vi "Remove by Name.vi"(8 "error in (no error)":errorcluster, 11 "buffer_name":string="/example") -> (0 "error out":errorcluster)   [LabVIEW 2021, in "CIF_NI_CIPC.lvlib"]
doc: "Removes a CIPC buffer from the system."
uses:
  CIF_NI_CIPC.lvlib
  <vilib>/Utility/error.llb/Trim Whitespace.vi
  <vilib>/Utility/error.llb/Error Cluster From Error Code.vi
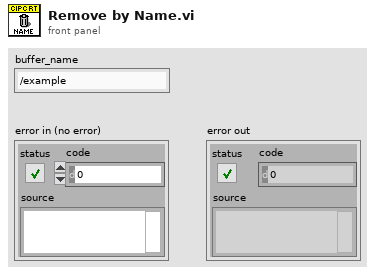
[diagram p1: front panel]
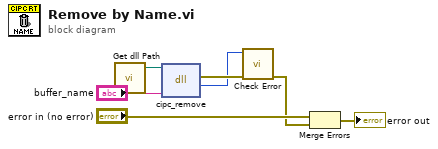
[diagram p0: block diagram]
diagram:
  n1 = call "Get dll Path.vi"() -> ("appended path"=w1:path)  [unwired: 5 in]
  n2 = dll-call lib="libnicipc.*" fn="cipc_remove"(path in=w1, "name"="buffer_name") -> (error out=w7:errorcluster, "return type"=w6:i32)  [unwired: 3 in, 1 out]
  n3 = call "Check Error.vi"("error in (no error)"=w7, "Error Code"=w6) -> ("error out"=w3:errorcluster)  [unwired: 9 in]
  n4 = Merge Errors("error in (no error)", w3) -> (→"error out":errorcluster)
